vi "Correlate Balls.vi"(10 "balls new":T1[](array[typedef]), 11 "balls":T1[](array[typedef])) -> (3 "balls new out":T1[](array[typedef]))   [LabVIEW 2016]
uses:
  SSL Detection Ball.ctl
  <vilib>/Analysis/Matrix/Datatypes/RealMatrix.ctl
  <vilib>/Analysis/Matrix/NI_Matrix.lvlib
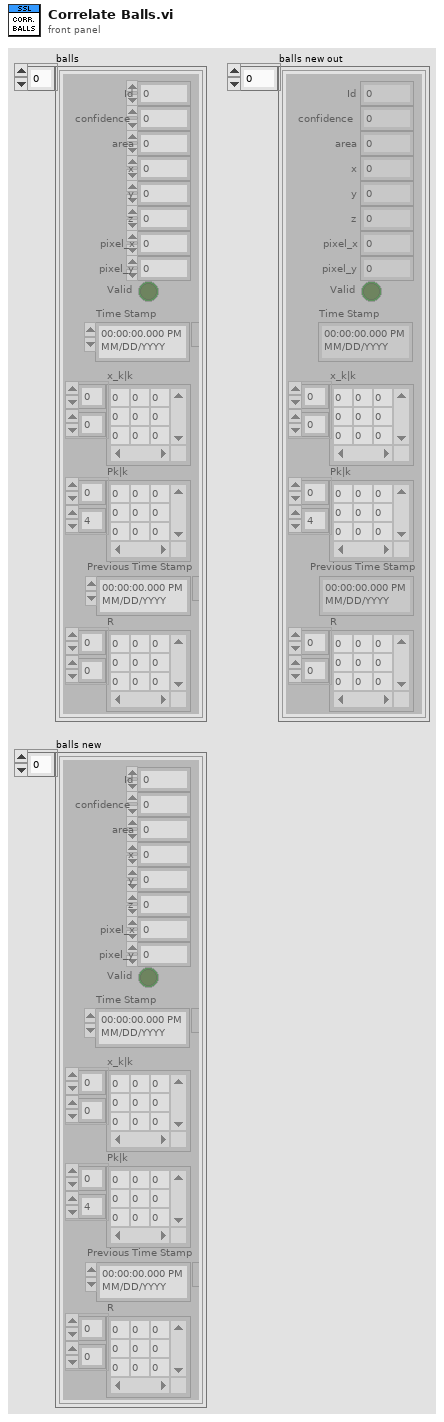
[diagram p1: front panel]
types:
  T1 = typedef "SSL Detection Ball.ctl" = cluster{"x":sgl, "area":u32, "confidence":sgl, "y":sgl, "z":sgl, "pixel_x":sgl, "pixel_y":sgl, "Valid":bool, "Time Stamp":timestamp, "x_k|k":T2, "Pk|k":T2, "Id":u32, "Previous Time Stamp":timestamp, "R":T2}
  T2 = typedef "NI_Matrix.lvlib/RealMatrix.ctl" = dbl[][]
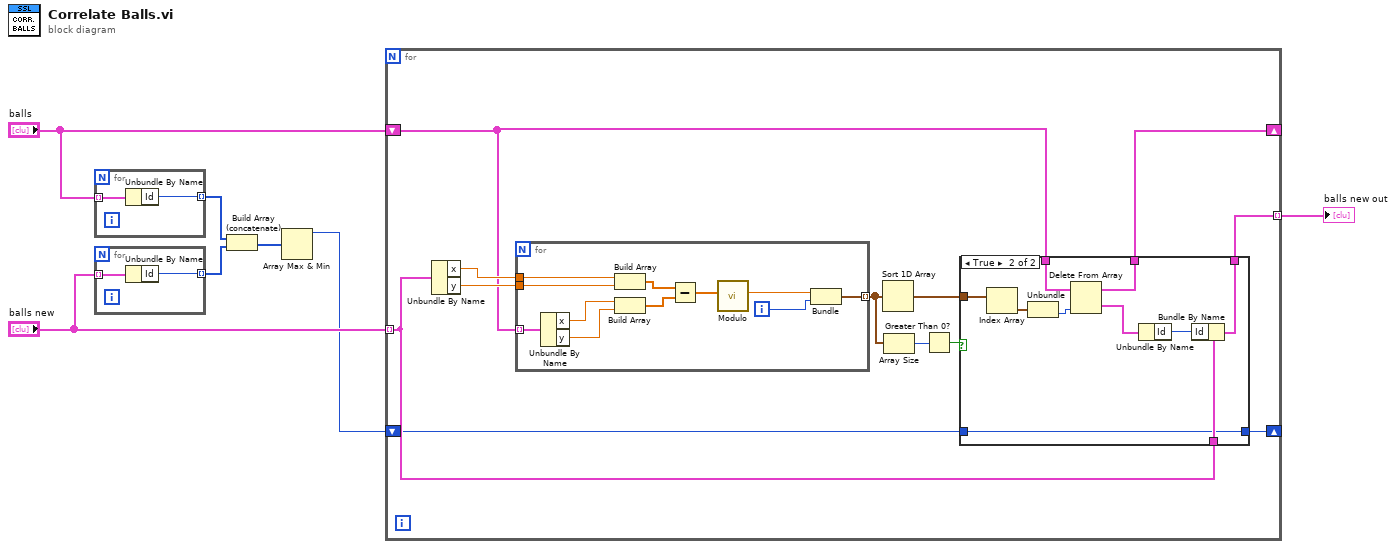
[diagram p0: block diagram]
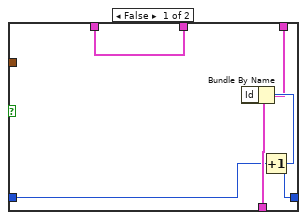
[diagram p2: hidden frame]
diagram:
  n1 = for {
    tunnel: "balls" -> [w9] mode=indexing
    tunnel: [w8] -> w5 mode=indexing
    n2 = Unbundle By Name(w9) -> ("Id"=w8:u32)
  }
  n3 = for {
    tunnel: "balls new" -> [w11] mode=indexing
    tunnel: [w10] -> w4 mode=indexing
    n4 = Unbundle By Name(w11) -> ("Id"=w10:u32)
  }
  n5 = Build Array (concatenate)(w5, w4) -> (w3:u32[])
  n6 = Array Max & Min(array=w3) -> (max value=w2:u32)  [unwired: 3 out]
  n7 = for {
    tunnel: "balls new" -> [w19] mode=indexing
    tunnel: [w17] -> w1 mode=indexing
    shift-right: [w18] -> _
    shift-left: "balls" -> [w21]
    shift-right: [w12] -> _
    shift-left: w2 -> [w13]
    n8 = Unbundle By Name(w19) -> ("x"=w23:sgl, "y"=w22:sgl)
    n9 = for {
      tunnel: w23 -> [w49]
      tunnel: w22 -> [w48]
      tunnel: w21 -> [w45] mode=indexing
      tunnel: [w39] -> w16 mode=indexing
      i -> [w40]
      n10 = Unbundle By Name(w45) -> ("x"=w44:sgl, "y"=w43:sgl)
      n11 = Build Array(w49, w48) -> (w47:sgl[])
      n12 = Build Array(w44, w43) -> (w42:sgl[])
      n13 = Subtract(x=w47, y=w42) -> (x-y=w46:sgl[])
      n14 = call "Modulo.vi"("2D vector"=w46) -> ("Modulo"=w41:dbl)  [unwired: 10 in]
      n15 = Bundle("Modulo"=w41, w40) -> (w39:cluster{"Modulo":dbl, i32})  [unwired: 1 in]
    }
    n16 = Sort 1D Array(array=w16) -> (sorted array=w20:cluster{"Modulo":dbl, i32}[])
    n17 = Array Size(array=w16) -> (size(s)=w15:i32)
    n18 = Greater Than 0?(x=w15) -> (x > 0?=w14:bool)
    n19 = case shown="True" w14 {
      tunnel: w21 -> [w28 w38]
      tunnel: w20 -> [_ w37]
      tunnel: w19 -> [w27 w34]
      tunnel: [w28 w33] -> w18
      tunnel: [w24 w29] -> w17
      tunnel: w13 -> [w26 w30]
      tunnel: [w25 w30] -> w12
      frame False {
        n20 = Bundle By Name(cluster=w27, "Id"=w26) -> (w24:T1)
        n21 = Increment(x=w26) -> (x+1=w25:u32)
      }
      frame True {
        n22 = Index Array(array=w37) -> (element=w36:cluster{"Modulo":dbl, i32})  [unwired: 1 in]
        n23 = Unbundle(w36) -> (w35:i32)  [unwired: 1 out]
        n24 = Delete From Array(array=w38, index=w35) -> (deleted portion=w32:T1, array with subset deleted=w33:T1[])  [unwired: 1 in]
        n25 = Unbundle By Name(w32) -> ("Id"=w31:u32)
        n26 = Bundle By Name(cluster=w34, "Id"=w31) -> (w29:T1)
      }
    }
  }
  "balls new out" <- w1
